vi "Exercise 4-1.vi"(8 "error in (no error)":errorcluster, 9 "Min Temp":dbl, 10 "Max Temp":dbl, 11 "Current Temp":dbl) -> (1 "error out":errorcluster, 2 "Warning Text":string, 3 "Warning?":bool)   [LabVIEW 2014]
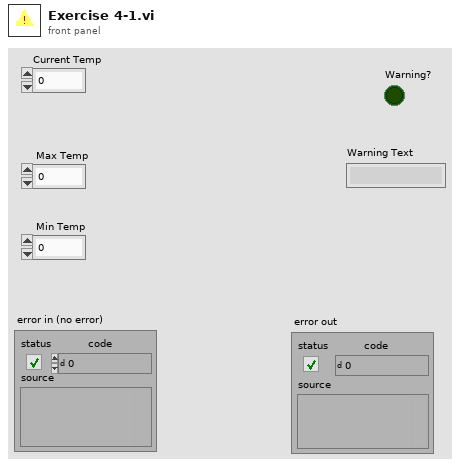
[diagram p1: front panel]
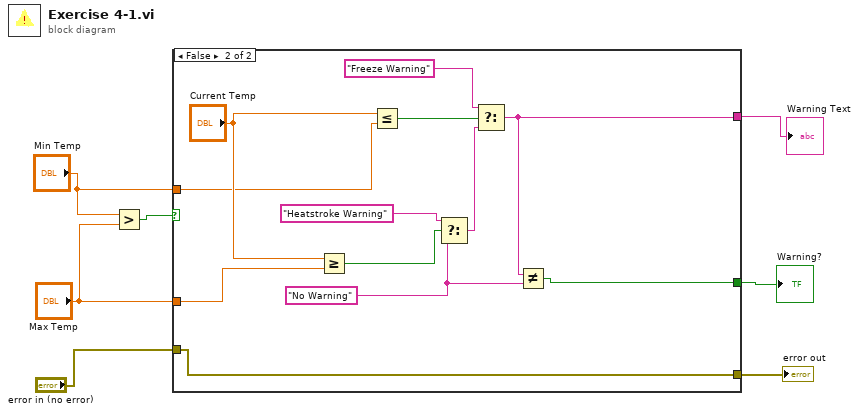
[diagram p0: block diagram]
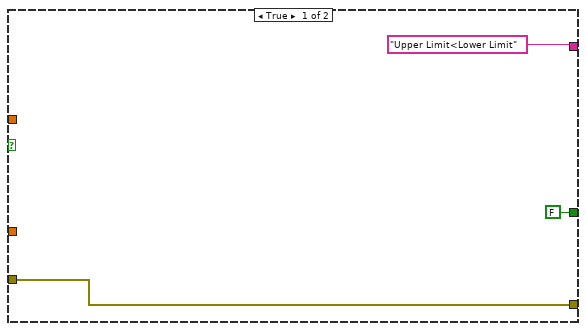
[diagram p2: hidden frame]
diagram:
  n1 = Greater?(x="Min Temp", y="Max Temp") -> (0:w7:bool)
  n2 = case shown="False" w7 {
    tunnel: "Max Temp" -> [_ w15]
    tunnel: "Min Temp" -> [_ w14]
    tunnel: ["Upper Limit<Lower Limit" w13] -> w4
    tunnel: [FALSE w12] -> w3
    tunnel: [w8 w11] -> w2
    tunnel: "error in (no error)" -> [w8 w11]
    frame True {
    }
    frame False {
      w16 = "No Warning"
      n3 = Greater Or Equal?(x="Current Temp", y=w15) -> (x >= y?=w21:bool)
      n4 = Less Or Equal?(x="Current Temp", y=w14) -> (x <= y?=w19:bool)
      n5 = Select(t="Heatstroke Warning", s=w21, f=w16) -> (s? t:f=w18:string)
      n6 = Select(t="Freeze Warning", s=w19, f=w18) -> (s? t:f=w13:string)
      n7 = Not Equal?(x=w13, y=w16) -> (x != y?=w12:bool)
    }
  }
  "Warning Text" <- w4
  "Warning?" <- w3
  "error out" <- w2
